vi "Add Byte.vi"(8 "error in":errorcluster, 10 "byte":u8 format="%02x", 11 "Buffer":refnum<data-value>) -> (0 "error out":errorcluster, 3 "Buffer":refnum<data-value>)   [LabVIEW 2013, in "ByteBuffer.lvclass"]
doc: "This VI writes one data element into the current location in the buffer. The location in the buffer is updated automatically."
uses:
  ByteBuffer.lvclass
  VariantBuffer/VariantBuffer.lvclass
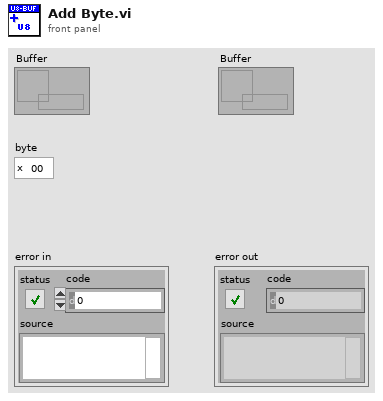
[diagram p1: front panel]
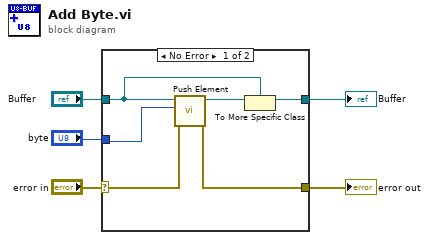
[diagram p0: block diagram]
diagram:
  n1 = case shown="No Error" "error in" {
    selector: "error in" -> [w9 w13]
    tunnel: "Buffer" -> [w6 w12]
    tunnel: [w7 w12] -> w4
    tunnel: [w8 w13] -> w3
    tunnel: "byte" -> [w11 _]
    frame No Error {
      n2 = call "Push Element.vi"("error in"=w9, "element"=w11, "Buffer in"=w6) -> ("error out"=w8:errorcluster, "Buffer"=w10:refnum<data-value>)  [unwired: 7 in]
      n3 = To More Specific Class(target class=w6, reference=w10) -> (specific class reference=w7:refnum<data-value>)  [unwired: 1 in, 1 out]
    }
    frame Error {
    }
  }
  "error out" <- w3
  "Buffer" <- w4
